vi "Decode HydroHarp v1 TTT Data.vi"(8 "oflcorr_in":u64, 11 "rawbits":u32) -> (0 "oflcorr_out":u64, 1 "channel":u8, 2 "dtime":u32, 3 "truetime":u64, 4 "markercode":u32)   [LabVIEW 2021, in "PTU Files.lvlib"]
uses:
  PTU Files.lvlib
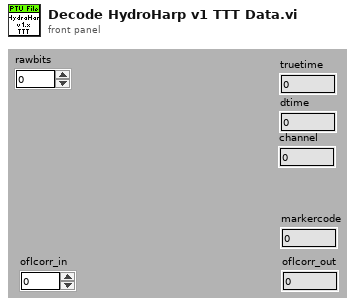
[diagram p1: front panel]
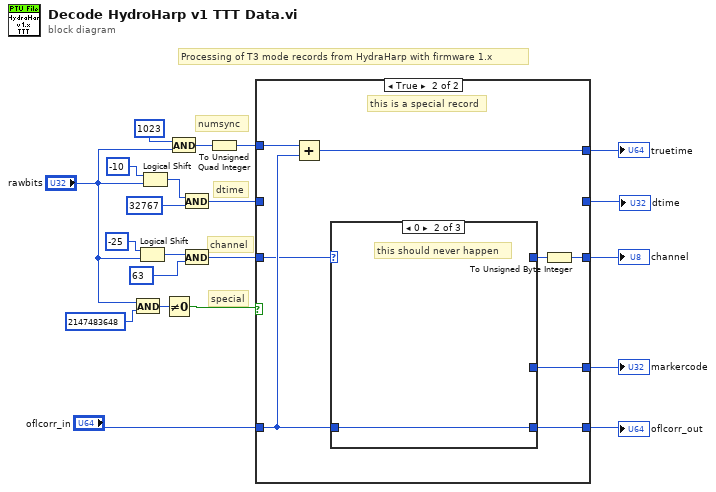
[diagram p0: block diagram]
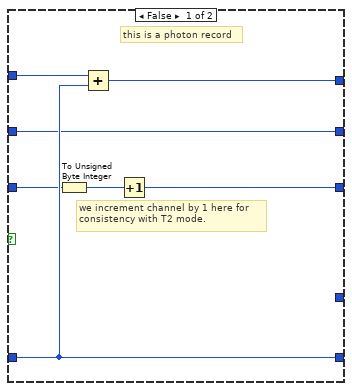
[diagram p2: hidden frame]
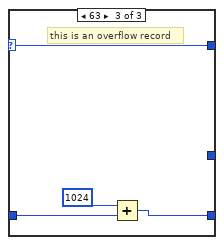
[diagram p4: hidden frame]
diagram:
  # "special"
  # "Processing of T3 mode records from HydraHarp with firmware 1.x"
  # "dtime"
  # "channel"
  # "numsync"
  n1 = And(x="rawbits", y=u32 2147483648 ("x")) -> (x .and. y?=w6:u32)
  n2 = Logical Shift(y=-25, x="rawbits") -> (x << y=w14:u32)
  n3 = Logical Shift(y=-10, x="rawbits") -> (x << y=w17:u32)
  n4 = Not Equal To 0?(x=w6) -> (x != 0?=w3:bool)
  n5 = And(x=u32 1023, y="rawbits") -> (x .and. y?=w19:u32)
  n6 = And(x=w17, y=u32 32767 ("x")) -> (x .and. y?=w15:u32)
  n7 = And(x=w14, y=u32 63 ("x")) -> (x .and. y?=w2:u32)
  n8 = To Unsigned Quad Integer(1:w19) -> (0:w1:u64)
  n9 = case shown="True" w3 {
    tunnel: w1 -> [w25 w36]
    tunnel: "oflcorr_in" -> [w28 w34]
    tunnel: [w28 w33] -> w11
    tunnel: [_ w32] -> w10
    tunnel: w15 -> [w26 _]
    tunnel: [w27 w35] -> w8
    tunnel: [w26 _] -> w7
    tunnel: [w23 w29] -> w9
    tunnel: w2 -> [w24 w31]
    frame False {
      # "we increment channel by 1 here for\nconsistency with T2 mode."
      # "this is a photon record"
      n10 = To Unsigned Byte Integer(number=w24) -> (unsigned 8bit integer=w22:u8)
      n11 = Add(x=w25, y=w28) -> (x+y=w27:u64)
      n12 = Increment(x=w22) -> (x+1=w23:u8)
    }
    frame True {
      # "this is a special record"
      n13 = Add(x=w36, y=w34) -> (x+y=w35:u64)
      n14 = case shown="0" w31 {
        selector: w31 -> [w37 _ w40]
        tunnel: w34 -> [w38 w39 w43]
        tunnel: [w38 w39 w42] -> w33
        tunnel: [w37 _ _] -> w32
        tunnel: [_ _ w40] -> w30
        frame Default {
          # "this is a marker record"
        }
        frame 0 {
          # "this should never happen"
        }
        frame 63 {
          # "this is an overflow record"
          n15 = Add(x=u64 1024, y=w43) -> (x+y=w42:u64)
        }
      }
      n16 = To Unsigned Byte Integer(number=w30) -> (unsigned 8bit integer=w29:u8)
    }
  }
  "channel" <- w9
  "truetime" <- w8
  "markercode" <- w10
  "oflcorr_out" <- w11
  "dtime" <- w7
